vi "File_to_UDcluster.vi"(0 "Cyphered text":string, 11 "error in (no error)":errorcluster) -> (4 "User-data cluster":T1, 15 "error out":errorcluster)   [LabVIEW 2012]
uses:
  typedef/User_Data_Cluster.ctl
  typedef/User Accounts.ctl
panel:
  in  "User-data type":T1
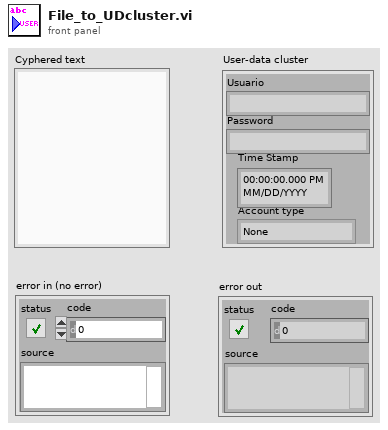
[diagram p1: front panel]
types:
  T1 = typedef "User_Data_Cluster.ctl" = cluster{"Usuario":string, "Password":string, "Account type":T2, "Time Stamp":timestamp}
  T2 = typedef "User Accounts.ctl" = enum16{"None", "User", "Admin"}
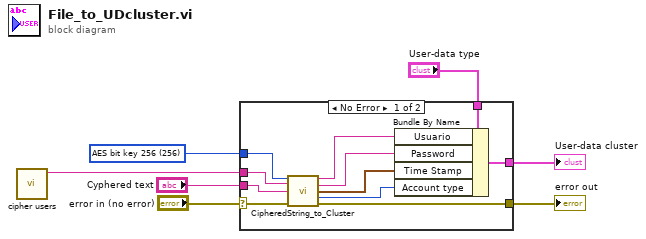
[diagram p0: block diagram]
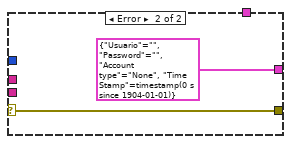
[diagram p2: hidden frame]
diagram:
  w3 = u16 256 items=["AES bit key 128"=128, "AES bit key 192"=192, "AES bit key 256"=256] ("BitKeyType (256)")
  n1 = call "cipher users.vi"() -> ("password to cipher users"=w4:string)  [unwired: 11 in]
  n2 = case shown="No Error" "error in (no error)" {
    selector: "error in (no error)" -> [w16 w20]
    tunnel: "Cyphered text" -> [w18 _]
    tunnel: [w17 T1 {"Usuario"="", "Password"="", "Account type"=enum."None", "Time Stamp"=timestamp(0 s since 1904-01-01)} ("User-data type out 2")] -> w7
    tunnel: [w15 w20] -> w5
    tunnel: w4 -> [w14 _]
    tunnel: w3 -> [w13 _]
    tunnel: "User-data type" -> [w12 _]
    frame No Error {
      n3 = call "CipheredString_to_Cluster.vi"("BitKeyType (256)"=w13, "password to cipher users"=w14, "Cyphered text"=w18, "error in (no error)"=w16) -> ("String 1"=w10:string, "String 2"=w11:string, "Time Stamp"=w8:timestamp, "Account"=w9:T2, "error out"=w15:errorcluster)  [unwired: 7 in]
      n4 = Bundle By Name(cluster=w12, "Usuario"=w10, "Password"=w11, "Time Stamp"=w8, "Account type"=w9) -> (w17:T1)
    }
    frame Error {
    }
  }
  "User-data cluster" <- w7
  "error out" <- w5
